vi "ControlePosicaoServo.vi"() -> ()   [LabVIEW 2012]
uses:
  <vilib>/LabVIEW Interface for Arduino/Type Defs/Board Type.ctl
  <vilib>/LabVIEW Interface for Arduino/Type Defs/Pin Mode.ctl
  <vilib>/Utility/file.llb/Read From Spreadsheet File (I64).vi
  <vilib>/LabVIEW Interface for Arduino/LabVIEW Interface for Arduino.lvlib
panel:
  out "first row":i64[](array[numeric])
  in  "Comeco do Arquivo":i32
  out "Elemento do Arquivo":i64
  in  "file path (dialog if empty)":path
  in  "TXT    KNOOB":bool
  out "PWM2":i32
  out "PWM1":i32
  out "Erro":dbl
  in  "Referencia":dbl(knob) scale=0.0..180.0
  out "Referencia":dbl(knob) scale=0.0..180.0
  in  "stop":bool
  out "Atual":dbl(knob) scale=0.0..180.0
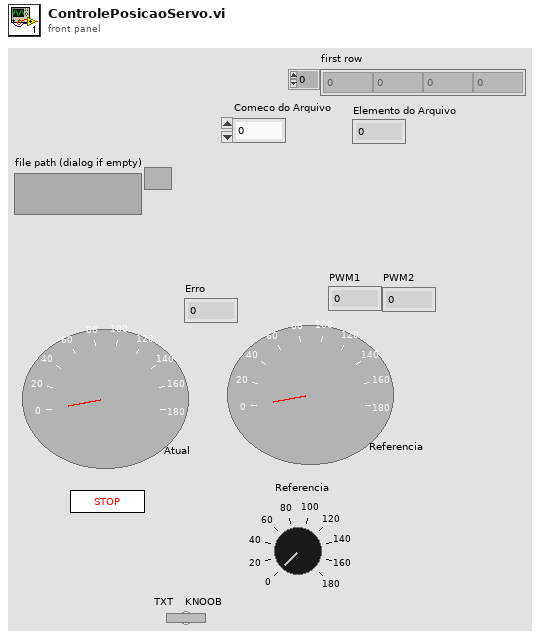
[diagram p1: front panel]
types:
  T1 = typedef "LabVIEW Interface for Arduino.lvlib/Board Type.ctl" = enum16{"Uno", "Dimuelanove w/Atmega 328", "Mega 2560"}
  T2 = typedef "LabVIEW Interface for Arduino.lvlib/Arduino Resource.ctl" = cluster{"VISA resource":refnum<visa-resource-name>, "Board Type":T1, "Connection Type":enum8{"USB / Serial"}, "Bytes Per Packet (15)":u8}
  T3 = typedef "LabVIEW Interface for Arduino.lvlib/Pin Mode.ctl" = enum8{"Input", "Output"}
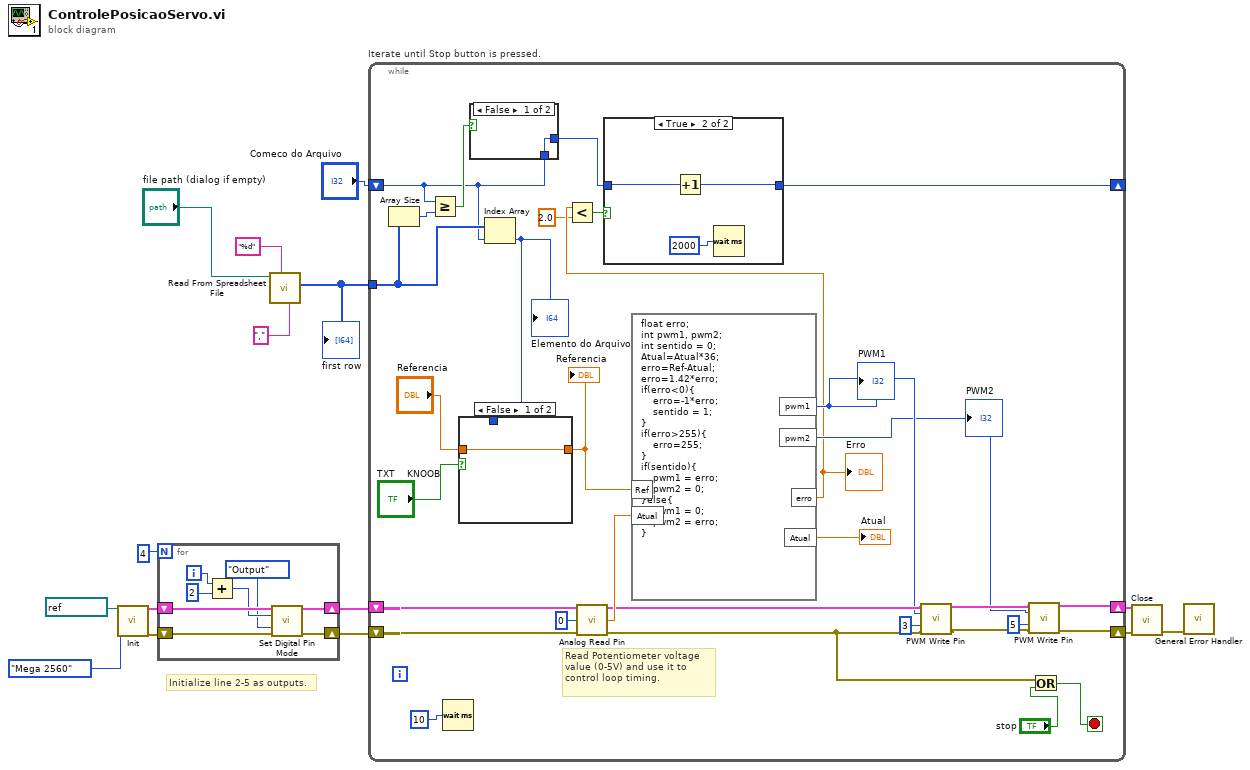
[diagram p0: block diagram]
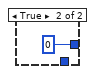
[diagram p2: hidden frame]
diagram:
  # "Initialize line 2-5 as outputs."
  n1 = call <vilib>:"Init.vi"("VISA resource"=refnum<visa-resource-name> "COM4", "Board Type (Uno)"=Board_Type."Mega 2560") -> ("Arduino Resource"=w14:T2, "error out"=w15:errorcluster)  [unwired: 16 in]
  n2 = for {
    N: 4 -> [_]
    shift-right: [w21] -> w11
    shift-left: w14 -> [w22]
    shift-right: [w20] -> w10
    shift-left: w15 -> [w23]
    i -> [w19]
    n3 = Add(x=w19, y=2) -> (x+y=w17:i32)
    n4 = call <vilib>:"Set Digital Pin Mode.vi"("Arduino Resource"=w22, "Digital I/O Pin"=w17, "Pin Mode (Input)"=Pin_Mode."Output", "error in"=w23) -> ("Arduino Resource"=w21:T2, "error out"=w20:errorcluster)  [unwired: 10 in]
  }
  n5 = call-poly <vilib>:"Read From Spreadsheet File.vi"("delimiter (\\t)"="," ("delimiter (\\t)"), "format (%d)"="%d", "file path (dialog if empty)"="file path (dialog if empty)") -> ("first row"=w2:i64[])  [unwired: 4 in, 4 out]
  "first row" <- w2
  n6 = while "Iterate until Stop button is pressed." {
    shift-right: [w45] -> w13
    shift-left: w11 -> [w53]
    shift-right: [w44] -> w12
    shift-left: w10 -> [w54]
    tunnel: w2 -> [w28]
    shift-right: [w33] -> _
    shift-left: "Comeco do Arquivo" -> [w24]
    stop <- w37 stop-if-true
    # "Read Potentiometer voltage value (0-5V) and use it to control loop timing."
    n7 = Array Size(array=w28) -> (size(s)=w27:i32)
    n8 = Greater Or Equal?(x=w24, y=w27) -> (x >= y?=w25:bool)
    n9 = Wait (ms)(milliseconds to wait=u32 10) -> ()  [unwired: 1 out]
    n10 = case shown="False" w25 {
      tunnel: [w55 u32 0 ("milliseconds to wait")] -> w26
      tunnel: w24 -> [w55 _]
      frame False {
      }
      frame True {
      }
    }
    n11 = Index Array(array=w28, index=w24) -> (element=w32:i64)
    "Elemento do Arquivo" <- w32
    n12 = case shown="False" "TXT    KNOOB" {
      tunnel: "Referencia" -> [w57 _]
      tunnel: [w57 w58] -> w34
      tunnel: w32 -> [_ w58]
      frame False {
      }
      frame True {
      }
    }
    "Referencia" <- w34
    n13 = call <vilib>:"Analog Read Pin.vi"("Arduino Resource"=w53, "Analog Input Pin (0)"=u8 0, "error in"=w54) -> ("Arduino Resource"=w49:T2, "Voltage"=w51:dbl, "error out"=w38:errorcluster)  [unwired: 10 in]
    n14 = formula code="float erro;\nint pwm1, pwm2;\nint sentido = 0;\nAtual=Atual*36;\nerro=Ref-Atual;\nerro=1.42*erro;\nif(erro<0){\n    erro=-1*erro;\n    sentido = 1;\n}\nif(erro>255){\n    erro=255;\n}\nif(sentido){\n    pwm1 = erro;\n    pwm2 = 0;\n}else{\n    pwm1 = 0;\n    pwm2 = erro;\n}"("Ref"=w34, "Atual"=w51) -> ("erro"=w30:dbl, "Atual"=→"Atual":dbl, "pwm1"=w42:i32, "pwm2"=w41:i32)
    "Erro" <- w30
    "PWM1" <- w42
    "PWM2" <- w41
    n15 = Less?(x=w30, y=2.0) -> (x < y?=w31:bool)
    n16 = case shown="True" w31 {
      tunnel: w26 -> [w59 w61]
      tunnel: [w59 w60] -> w33
      frame False {
      }
      frame True {
        n17 = Increment(x=w61) -> (x+1=w60:u32)
        n18 = Wait (ms)(milliseconds to wait=u32 2000) -> ()  [unwired: 1 out]
      }
    }
    n19 = call <vilib>:"PWM Write Pin.vi"("Arduino Resource"=w49, "Duty Cycle (0 - 255)"=w42, "PWM Pin (3)"=u8 3, "error in"=w38) -> ("Arduino Resource"=w47:T2, "error out"=w46:errorcluster)  [unwired: 10 in]
    n20 = call <vilib>:"PWM Write Pin.vi"("Arduino Resource"=w47, "Duty Cycle (0 - 255)"=w41, "PWM Pin (3)"=u8 5, "error in"=w46) -> ("Arduino Resource"=w45:T2, "error out"=w44:errorcluster)  [unwired: 10 in]
    n21 = Or(x=w38, y="stop") -> (x .or. y?=w37:bool)
  }
  n22 = call <vilib>:"Close.vi"("Arduino Resource"=w13, "error in"=w12) -> ("error out"=w7:errorcluster)  [unwired: 13 in]
  n23 = call <vilib>:"General Error Handler.vi"("error in (no error)"=w7) -> ()  [unwired: 10 in, 5 out]
